vi "Initialize Connection.vi"(8 "error in (no error)":errorcluster, 11 "Connection Reference In":refnum<data-value>) -> (0 "error out":errorcluster, 3 "Connection Reference Out":refnum<data-value>)   [LabVIEW 2020, in "Connection Reference.lvlib" / "Connection Reference.lvclass"]
uses:
  <vilib>/gpm_packages/@cs/Network-interface/Source/Connection Reference/Connection Reference/Connection Reference.lvclass
  <vilib>/gpm_packages/@cs/Network-interface/Source/Connection Reference/Connection Reference/Connection Reference.lvclass/Connection Reference.ctl
  <vilib>/gpm_packages/@cs/Network-interface/Source/Connection Reference/IConnection/IConnection.lvclass
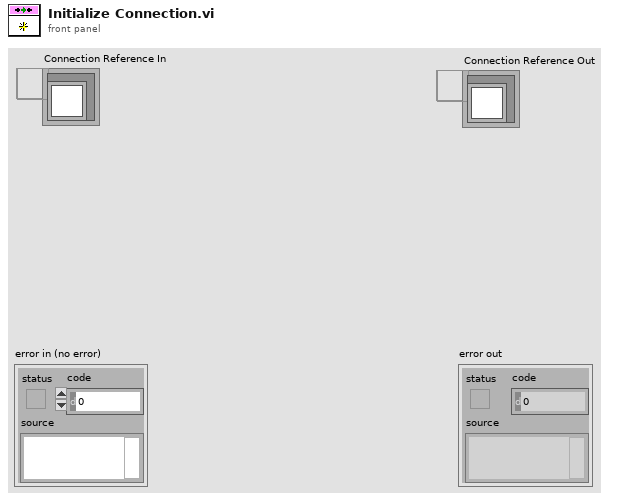
[diagram p1: front panel]
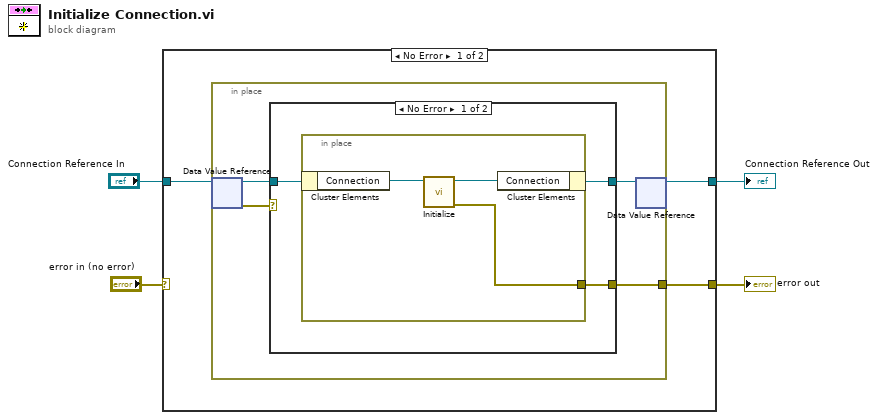
[diagram p0: block diagram]
diagram:
  n1 = case shown="No Error" "error in (no error)" {
    selector: "error in (no error)" -> [_ w20]
    tunnel: "Connection Reference In" -> [w7 w21]
    tunnel: [w6 w21] -> w3
    tunnel: [w5 w20] -> w1
    frame No Error {
      n2 = in-place {
        in-place-border: [w8] -> w5
        n3 = in-place-dvr #1(w7) -> (w11:refnum<class "Connection Reference.lvclass">, w9:errorcluster)
        n4 = case shown="No Error" w9 {
          selector: w9 -> [_ w18]
          tunnel: w11 -> [w14 w19]
          tunnel: [w13 w19] -> w10
          tunnel: [w12 w18] -> w8
          frame No Error {
            n5 = in-place {
              in-place-border: [w15] -> w12
              n6 = in-place-cluster #2(w14) -> ("Connection"=w17:refnum<class "IConnection.lvclass">)
              n7 = call-dynamic "Initialize.vi"("IConnection in"=w17) -> ("error out"=w15:errorcluster, "IConnection out"=w16:refnum<class "IConnection.lvclass">)  [unwired: 9 in]
              n8 = in-place-cluster #2("Connection"=w16) -> (w13:refnum<class "Connection Reference.lvclass">)
            }
          }
          frame Error {
            # "#todo add useful error here"
          }
        }
        n9 = in-place-dvr #1(w10) -> (w6:refnum<data-value>)  [unwired: 1 out]
      }
    }
    frame Error {
    }
  }
  "error out" <- w1
  "Connection Reference Out" <- w3
